vi "InsertDataDE.vi"(8 "error in":errorcluster, 11 "检测电极":T1) -> (0 "error out":errorcluster)   [LabVIEW 2014, in "DataBase.lvlib"]
uses:
  DataBase.lvlib
  <vilib>/addons/database/Connection.llb/DB Tools Open Connec (String).vi
  <vilib>/addons/database/Connection.llb/Conn Execute.vi
  <vilib>/addons/database/Recordset.llb/Rec Destroy - Connection.vi
  <vilib>/addons/database/NI_Database_API.lvlib
panel:
  in  "table":string
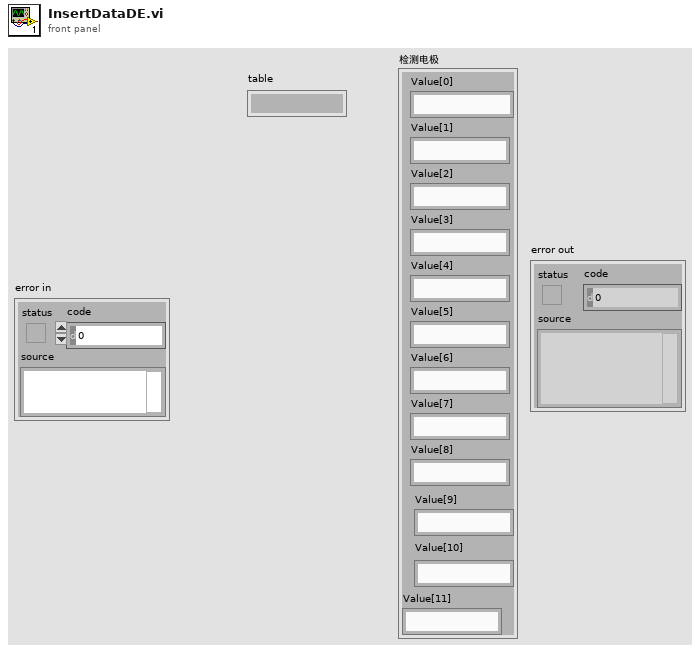
[diagram p1: front panel]
types:
  T1 = cluster{"Value[0]":string, "Value[1]":string, "Value[2]":string, "Value[3]":string, "Value[4]":string, "Value[5]":string, "Value[6]":string, "Value[7]":string, "Value[8]":string, "Value[9]":string, "Value[10]":string, "Value[11]":string}
  T2 = typedef "NI_Database_API.lvlib/Conn ObjectReference.ctl" = refnum<k1>
  T3 = typedef "NI_Database_API.lvlib/Rec ObjectReference.ctl" = refnum<k1>
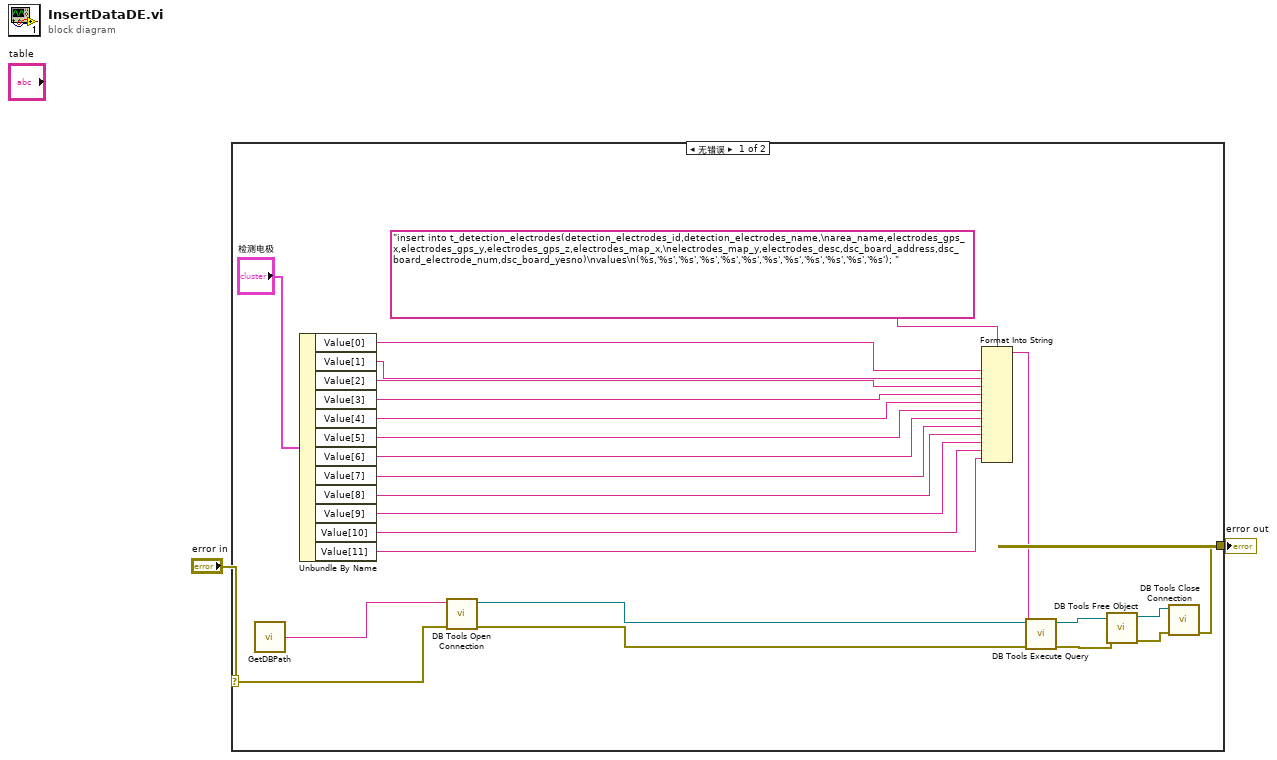
[diagram p0: block diagram]
diagram:
  n1 = case shown="无错误" "error in" {
    selector: "error in" -> [w22 w27]
    tunnel: [w21 w27] -> w1
    frame No Error {
      n2 = call "GetDBPath.vi"() -> ("Connection"=w20:string)  [unwired: 1 in]
      n3 = Unbundle By Name("检测电极") -> ("Value[0]"=w9:string, "Value[1]"=w10:string, "Value[2]"=w11:string, "Value[3]"=w12:string, "Value[4]"=w13:string, "Value[5]"=w14:string, "Value[6]"=w15:string, "Value[7]"=w16:string, "Value[8]"=w17:string, "Value[9]"=w5:string, "Value[10]"=w4:string, "Value[11]"=w3:string)
      n4 = call-poly <vilib>:"DB Tools Open Connection.vi"("error in (no error)"=w22, "connection information"=w20) -> ("error out"=w25:errorcluster, "connection reference"=w26:T2)  [unwired: 6 in]
      n5 = Format Into String(format string="insert into t_detection_electrodes(detection_electrodes_id,detection_electrodes_name,\narea_name,electrodes_gps_x,electrodes_gps_y,electrodes_gps_z,electrodes_map_x,\nelectrodes_map_y,electrodes_desc,dsc_board_address,dsc_board_electrode_num,dsc_board_yesno)\nvalues\n(%s,'%s','%s','%s','%s','%s','%s','%s','%s','%s','%s','%s'); ", w9, w10, w11, w12, w13, w14, w15, w16, w17, w5, w4, w3) -> (resulting string=w6:string)  [unwired: 2 in, 1 out]
      n6 = call-poly <vilib>:"DB Tools Execute Query.vi"("error in (no error)"=w25, "SQL query"=w6, "connection reference"=w26) -> ("error out"=w18:errorcluster, "recordset reference"=w19:T3)  [unwired: 5 in]
      n7 = call-poly <vilib>:"DB Tools Free Object.vi"("error in (no error)"=w18, "recordset reference"=w19) -> ("error out"=w24:errorcluster, "connection reference"=w23:T2)  [unwired: 8 in]
      n8 = call <vilib>:"DB Tools Close Connection.vi"("error in (no error)"=w24, "connection reference"=w23) -> ("error out"=w21:errorcluster)  [unwired: 5 in]
    }
    frame Error {
    }
  }
  "error out" <- w1
